vi "Do.vi"(8 "error in":errorcluster, 10 "Actor in":refnum<class "Actor.lvclass">, 11 "Save Main File MSG":refnum<class "Save Main File MSG.lvclass">) -> (0 "error out":errorcluster, 2 "Actor out":refnum<class "Actor.lvclass">)   [LabVIEW 2014, in "Controller.lvlib" / "Save Main File MSG.lvclass"]
doc: "(<B>Filename</B>: Actor Framework.lvlib:Message.lvclass:Do.vi)\n\nDefines what a message does when it is received by an actor. Generally, a message instructs an actor to invoke one of its methods. By default, this method does nothing. A child class must override it to define behavior. Create a child class by using the Actor Framework Message Maker dialog box."
uses:
  Save Main File MSG.lvclass
  <vilib>/ActorFramework/Actor/Actor.lvclass
  File Actor/Messages/Abstract/Saving File Message/Saving File Message.lvclass/Saving File Message.ctl
  Controller.lvclass
  SuperActor/SuperClass.lvclass/SuperClass.ctl
  File Actor/Messages/Abstract/Saving File Message/Read Saving.vi
  SuperActor/Read Log Session.vi
  <userlib>/_Session Fwk/Session - Root.lvclass
  <vilib>/NI_Real-Time Target Support.lvlib
  reusable/Session APIs/Session Log/System Log.lvclass
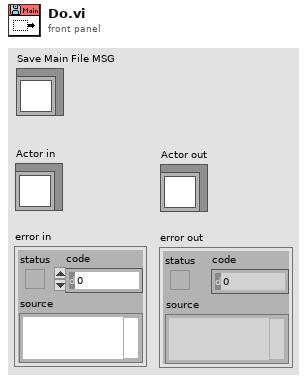
[diagram p1: front panel]
types:
  T1 = typedef "Session - Root.lvclass/Session Handle.ctl" = refnum<data-value>
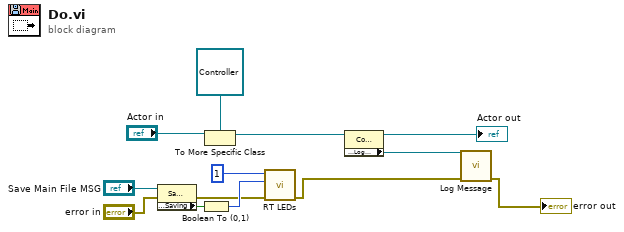
[diagram p0: block diagram]
diagram:
  n1 = property class="Save Main File MSG"(reference="Save Main File MSG", error in="error in") -> (error out=w8:errorcluster, "Accessors:Saving"=w12:bool)  [unwired: 1 out]
  n2 = Boolean To (0,1)(Boolean=w12) -> (0, 1=w10:i16)
  n3 = To More Specific Class(target class=refnum<class "Controller.lvclass"> refnum ("Controller:Controller"), reference="Actor in") -> (specific class reference=w5:refnum<class "Controller.lvclass">)  [unwired: 1 in, 1 out]
  n4 = call <vilib>:"RT LEDs.vi"("error in (no error)"=w8, "State"=w10, "LED Num"=1) -> ("error out"=w2:errorcluster)  [unwired: 3 in, 1 out]
  n5 = property class="Controller"(reference=w5) -> (reference out=→"Actor out":refnum<class "Controller.lvclass">, "Accessors:Log Session"=w3:T1)  [unwired: 1 in, 1 out]
  n6 = call "Log Message.vi"("error in"=w2, "session in"=w3) -> ("error out"=→"error out":errorcluster)  [unwired: 8 in, 1 out]
